vi "App Time format.vi"() -> (8 "App timeformat":string="%<%Y.%m.%d %H:%M:%S>T")   [LabVIEW 2011]
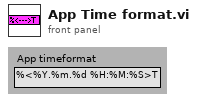
[diagram p1: front panel]
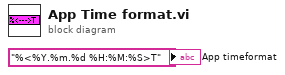
[diagram p0: block diagram]
diagram:
  "App timeformat" <- "%<%Y.%m.%d %H:%M:%S>T"
